vi "Queue destroy.vi"(11 "output cluster":T1) -> (3 "error out":errorcluster)   [LabVIEW 2015]
uses:
  QMH Fundamentals - Message Cluster.ctl
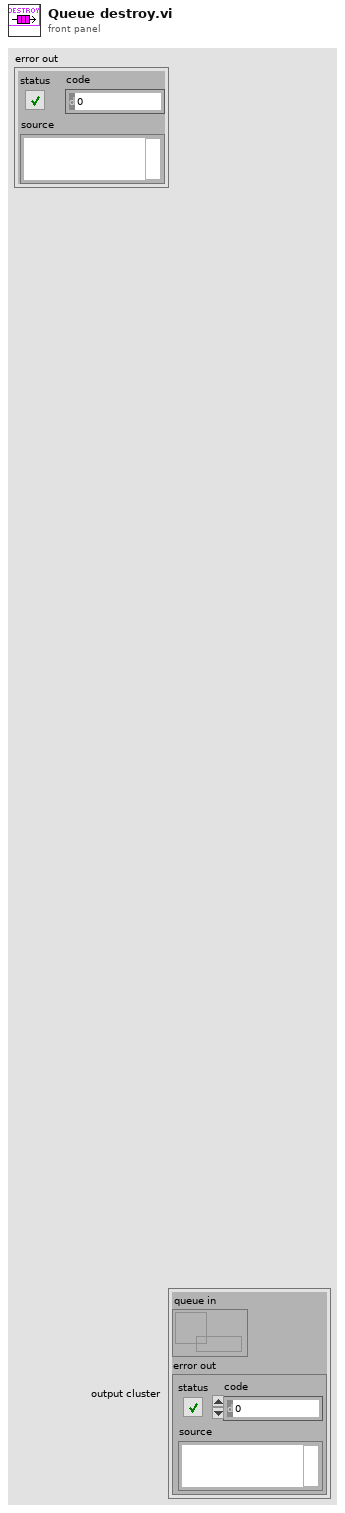
[diagram p1: front panel]
types:
  T1 = cluster{"queue in":refnum<queue>, "error out":errorcluster}
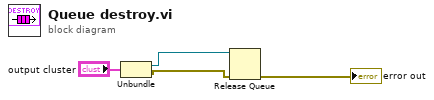
[diagram p0: block diagram]
diagram:
  n1 = Unbundle("output cluster") -> ("queue in"=w2:refnum<queue>, "error out"=w1:errorcluster)
  n2 = Release Queue(queue=w2, error in (no error)=w1) -> (error out=→"error out":errorcluster)  [unwired: 1 in, 2 out]
